vi "USB3 Get Camera Info.vi"(8 "error in (no error)":errorcluster, 10 "pCameraInfo":T1, 11 "ulIndex":u32) -> (0 "error out":errorcluster, 2 "pCameraInfo out":T1, 3 "function return":i32)   [LabVIEW 2013, in "Octoplus_LIDAR.lvlib"]
doc: "CAMCMOSOCTUSB3_API int __cdecl USB3_GetCameraInfo(unsigned long ulIndex, tCameraInfo * pCameraInfo);"
uses:
  <userlib>/Octoplus_LIDAR/Octoplus_LIDAR.lvlib
  <userlib>/Octoplus_LIDAR/CamCmosOctUsb3.dll
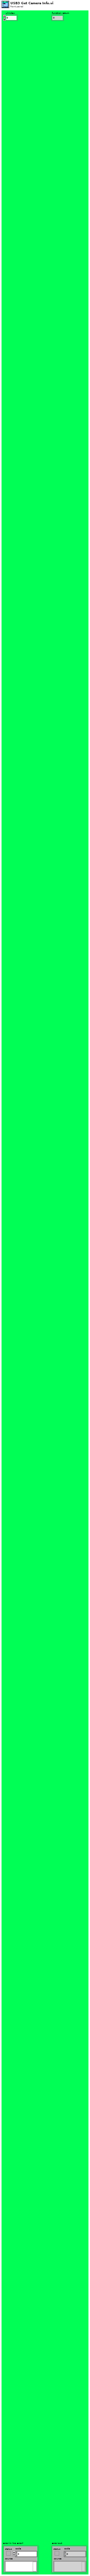
[diagram p1: front panel]
types:
  T1 = cluster{"pcID[0]":i8, "pcID[1]":i8, "pcID[2]":i8, "pcID[3]":i8, "pcID[4]":i8, "pcID[5]":i8, "pcID[6]":i8, "pcID[7]":i8, "pcID[8]":i8, "pcID[9]":i8, "pcID[10]":i8, "pcID[11]":i8, "pcID[12]":i8, "pcID[13]":i8, "pcID[14]":i8, "pcID[15]":i8, "pcID[16]":i8, "pcID[17]":i8, "pcID[18]":i8, "pcID[19]":i8, "pcID[20]":i8, "pcID[21]":i8, "pcID[22]":i8, "pcID[23]":i8, "pcID[24]":i8, "pcID[25]":i8, "pcID[26]":i8, "pcID[27]":i8, "pcID[28]":i8, "pcID[29]":i8, "pcID[30]":i8, "pcID[31]":i8, "pcID[32]":i8, "pcID[33]":i8, "pcID[34]":i8, "pcID[35]":i8, "pcID[36]":i8, "pcID[37]":i8, "pcID[38]":i8, "pcID[39]":i8, "pcID[40]":i8, "pcID[41]":i8, "pcID[42]":i8, "pcID[43]":i8, "pcID[44]":i8, "pcID[45]":i8, "pcID[46]":i8, "pcID[47]":i8, "pcID[48]":i8, "pcID[49]":i8, "pcID[50]":i8, "pcID[51]":i8, "pcID[52]":i8, "pcID[53]":i8, "pcID[54]":i8, "pcID[55]":i8, "pcID[56]":i8, "pcID[57]":i8, "pcID[58]":i8, "pcID[59]":i8, "pcID[60]":i8, "pcID[61]":i8, "pcID[62]":i8, "pcID[63]":i8, "pcID[64]":i8, "pcID[65]":i8, "pcID[66]":i8, "pcID[67]":i8, "pcID[68]":i8, "pcID[69]":i8, "pcID[70]":i8, "pcID[71]":i8, "pcID[72]":i8, "pcID[73]":i8, "pcID[74]":i8, "pcID[75]":i8, "pcID[76]":i8, "pcID[77]":i8, "pcID[78]":i8, "pcID[79]":i8, "pcID[80]":i8, "pcID[81]":i8, "pcID[82]":i8, "pcID[83]":i8, "pcID[84]":i8, "pcID[85]":i8, "pcID[86]":i8, "pcID[87]":i8, "pcID[88]":i8, "pcID[89]":i8, "pcID[90]":i8, "pcID[91]":i8, "pcID[92]":i8, "pcID[93]":i8, "pcID[94]":i8, "pcID[95]":i8, "pcID[96]":i8, "pcID[97]":i8, "pcID[98]":i8, "pcID[99]":i8, "pcID[100]":i8, "pcID[101]":i8, "pcID[102]":i8, "pcID[103]":i8, "pcID[104]":i8, "pcID[105]":i8, "pcID[106]":i8, "pcID[107]":i8, "pcID[108]":i8, "pcID[109]":i8, "pcID[110]":i8, "pcID[111]":i8, "pcID[112]":i8, "pcID[113]":i8, "pcID[114]":i8, "pcID[115]":i8, "pcID[116]":i8, "pcID[117]":i8, "pcID[118]":i8, "pcID[119]":i8, "pcID[120]":i8, "pcID[121]":i8, "pcID[122]":i8, "pcID[123]":i8, "pcID[124]":i8, "pcID[125]":i8, "pcID[126]":i8, "pcID[127]":i8, "pcID[128]":i8, "pcID[129]":i8, "pcID[130]":i8, "pcID[131]":i8, "pcID[132]":i8, "pcID[133]":i8, "pcID[134]":i8, "pcID[135]":i8, "pcID[136]":i8, "pcID[137]":i8, "pcID[138]":i8, "pcID[139]":i8, "pcID[140]":i8, "pcID[141]":i8, "pcID[142]":i8, "pcID[143]":i8, "pcID[144]":i8, "pcID[145]":i8, "pcID[146]":i8, "pcID[147]":i8, "pcID[148]":i8, "pcID[149]":i8, "pcID[150]":i8, "pcID[151]":i8, "pcID[152]":i8, "pcID[153]":i8, "pcID[154]":i8, "pcID[155]":i8, "pcID[156]":i8, "pcID[157]":i8, "pcID[158]":i8, "pcID[159]":i8, "pcID[160]":i8, "pcID[161]":i8, "pcID[162]":i8, "pcID[163]":i8, "pcID[164]":i8, "pcID[165]":i8, "pcID[166]":i8, "pcID[167]":i8, "pcID[168]":i8, "pcID[169]":i8, "pcID[170]":i8, "pcID[171]":i8, "pcID[172]":i8, "pcID[173]":i8, "pcID[174]":i8, "pcID[175]":i8, "pcID[176]":i8, "pcID[177]":i8, "pcID[178]":i8, "pcID[179]":i8, "pcID[180]":i8, "pcID[181]":i8, "pcID[182]":i8, "pcID[183]":i8, "pcID[184]":i8, "pcID[185]":i8, "pcID[186]":i8, "pcID[187]":i8, "pcID[188]":i8, "pcID[189]":i8, "pcID[190]":i8, "pcID[191]":i8, "pcID[192]":i8, "pcID[193]":i8, "pcID[194]":i8, "pcID[195]":i8, "pcID[196]":i8, "pcID[197]":i8, "pcID[198]":i8, "pcID[199]":i8, "pcID[200]":i8, "pcID[201]":i8, "pcID[202]":i8, "pcID[203]":i8, "pcID[204]":i8, "pcID[205]":i8, "pcID[206]":i8, "pcID[207]":i8, "pcID[208]":i8, "pcID[209]":i8, "pcID[210]":i8, "pcID[211]":i8, "pcID[212]":i8, "pcID[213]":i8, "pcID[214]":i8, "pcID[215]":i8, "pcID[216]":i8, "pcID[217]":i8, "pcID[218]":i8, "pcID[219]":i8, "pcID[220]":i8, "pcID[221]":i8, "pcID[222]":i8, "pcID[223]":i8, "pcID[224]":i8, "pcID[225]":i8, "pcID[226]":i8, "pcID[227]":i8, "pcID[228]":i8, "pcID[229]":i8, "pcID[230]":i8, "pcID[231]":i8, "pcID[232]":i8, "pcID[233]":i8, "pcID[234]":i8, "pcID[235]":i8, "pcID[236]":i8, "pcID[237]":i8, "pcID[238]":i8, "pcID[239]":i8, "pcID[240]":i8, "pcID[241]":i8, "pcID[242]":i8, "pcID[243]":i8, "pcID[244]":i8, "pcID[245]":i8, "pcID[246]":i8, "pcID[247]":i8, "pcID[248]":i8, "pcID[249]":i8, "pcID[250]":i8, "pcID[251]":i8, "pcID[252]":i8, "pcID[253]":i8, "pcID[254]":i8, "pcID[255]":i8, "pcID[256]":i8, "pcID[257]":i8, "pcID[258]":i8, "pcID[259]":i8}
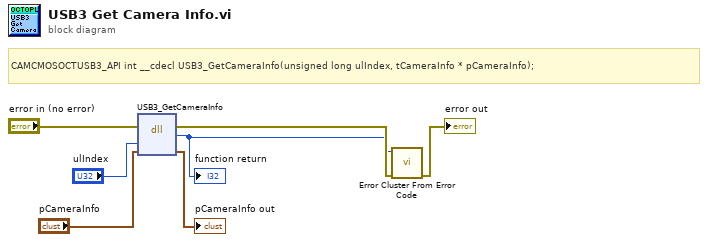
[diagram p0: block diagram]
diagram:
  # "CAMCMOSOCTUSB3_API int __cdecl USB3_GetCameraInfo(unsigned long ulIndex, tCameraInfo * pCameraInfo);"
  n1 = dll-call lib="C:/Program Files/National Instruments/LabVIEW 2013/user.lib/Octoplus_LIDAR/CamCmosOctUsb3.*" fn="USB3_GetCameraInfo"(error in="error in (no error)", "ulIndex"="ulIndex", "pCameraInfo"="pCameraInfo") -> (error out=w3:errorcluster, w1:i32, "pCameraInfo"=→"pCameraInfo out":T1)  [unwired: 3 in, 1 out]
  "function return" <- w1
  n2 = call <vilib>:"Error Cluster From Error Code.vi"("error in (no error)"=w3, "error code (0)"=w1) -> ("error out"=→"error out":errorcluster)  [unwired: 7 in]
